vi "File-Change Extension.vi"(0 "Path":path, 9 "new extension":string) -> (6 "new path":path)   [LabVIEW 2020]
panel:
  out "Path thru":path
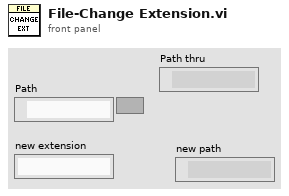
[diagram p1: front panel]
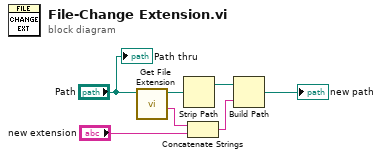
[diagram p0: block diagram]
diagram:
  n1 = call <vilib>:"Get File Extension.vi"("file"="Path") -> ("filename without extension"=w3:string, "dup file"=w2:path)  [unwired: 6 in, 3 out]
  n2 = Strip Path(path=w2) -> (stripped path=w5:path)  [unwired: 1 out]
  n3 = Concatenate Strings(w3, "new extension") -> (w6:string)
  n4 = Build Path(base path=w5, name or relative path=w6) -> (appended path=→"new path":path)
  "Path thru" <- "Path"
